vi "Basic Program Editor.vi"() -> ()   [LabVIEW 2012]
doc: "A stand alone program that can be used to quickly write and edit an OpenCL kernel. This program is not meant to be used except as a stand alone program. \n\n<b>Warning: This program calls OpenCLV Start.vi and OpenCLV Stop.vi and if used with other OpenCLV VIs may inadvertently delete devices and memory!</b>"
uses:
  Non-User VIs/Error Checking/Set Quiet Mode Functional Global.vi
  OpenCLV x64.lvlib
panel:
  out "Error Out":errorcluster
  # "Stand alone kernel editor.  Just run me \nto start creating OpenCL kernels!"
  # "Warning: I call OpenCLV Start.vi and OpenCLV Stop.vi \nif used with other OpenCLV VI's may delete device\nand memory!"
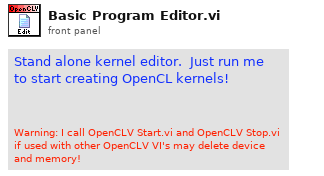
[diagram p1: front panel]
types:
  T1 = typedef "OpenCLV x64.lvlib/Device ID.ctl" = u64
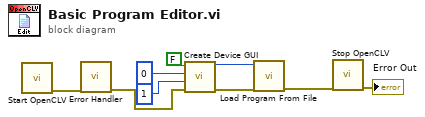
[diagram p0: block diagram]
diagram:
  n1 = call "Start OpenCLV.vi"() -> ("Error Out"=w2:errorcluster)  [unwired: 11 in]
  n2 = call-poly "Error Handler.vi"("Error In"=w2) -> ("Error Out"=w1:errorcluster)  [unwired: 10 in]
  n3 = call "Create Device GUI.vi"("Error In"=w1, "Device"=1, "Platform"=0, "Skip Configuration"=FALSE) -> ("error constant"=w5:errorcluster, "Device Reference"=w6:T1)  [unwired: 6 in]
  n4 = call "Load Program From File.vi"("Error In"=w5, "Device In"=w6) -> ("Error Out"=w4:errorcluster)  [unwired: 7 in, 2 out]
  n5 = call "Stop OpenCLV.vi"("Error In"=w4) -> ("Error Out"=→"Error Out":errorcluster)  [unwired: 10 in]
